vi "generate var cluster.vi"(8 "speed divider":dbl=1.0, 11 "Units":string(combo)) -> (0 "numarray":dbl[](array[numeric]), 1 "varnames":string[](array[string]), 2 "totarray":string[](array[string]), 3 "varclusterarray":T1(array[cluster]))   [LabVIEW 2017]
panel:
  out "Power":dbl[](array[numeric])
  out "appended array":dbl[](array[numeric])
  out "array w/ subset deleted":dbl[](array[numeric])
  out "String Array From File":string[][](array[string])
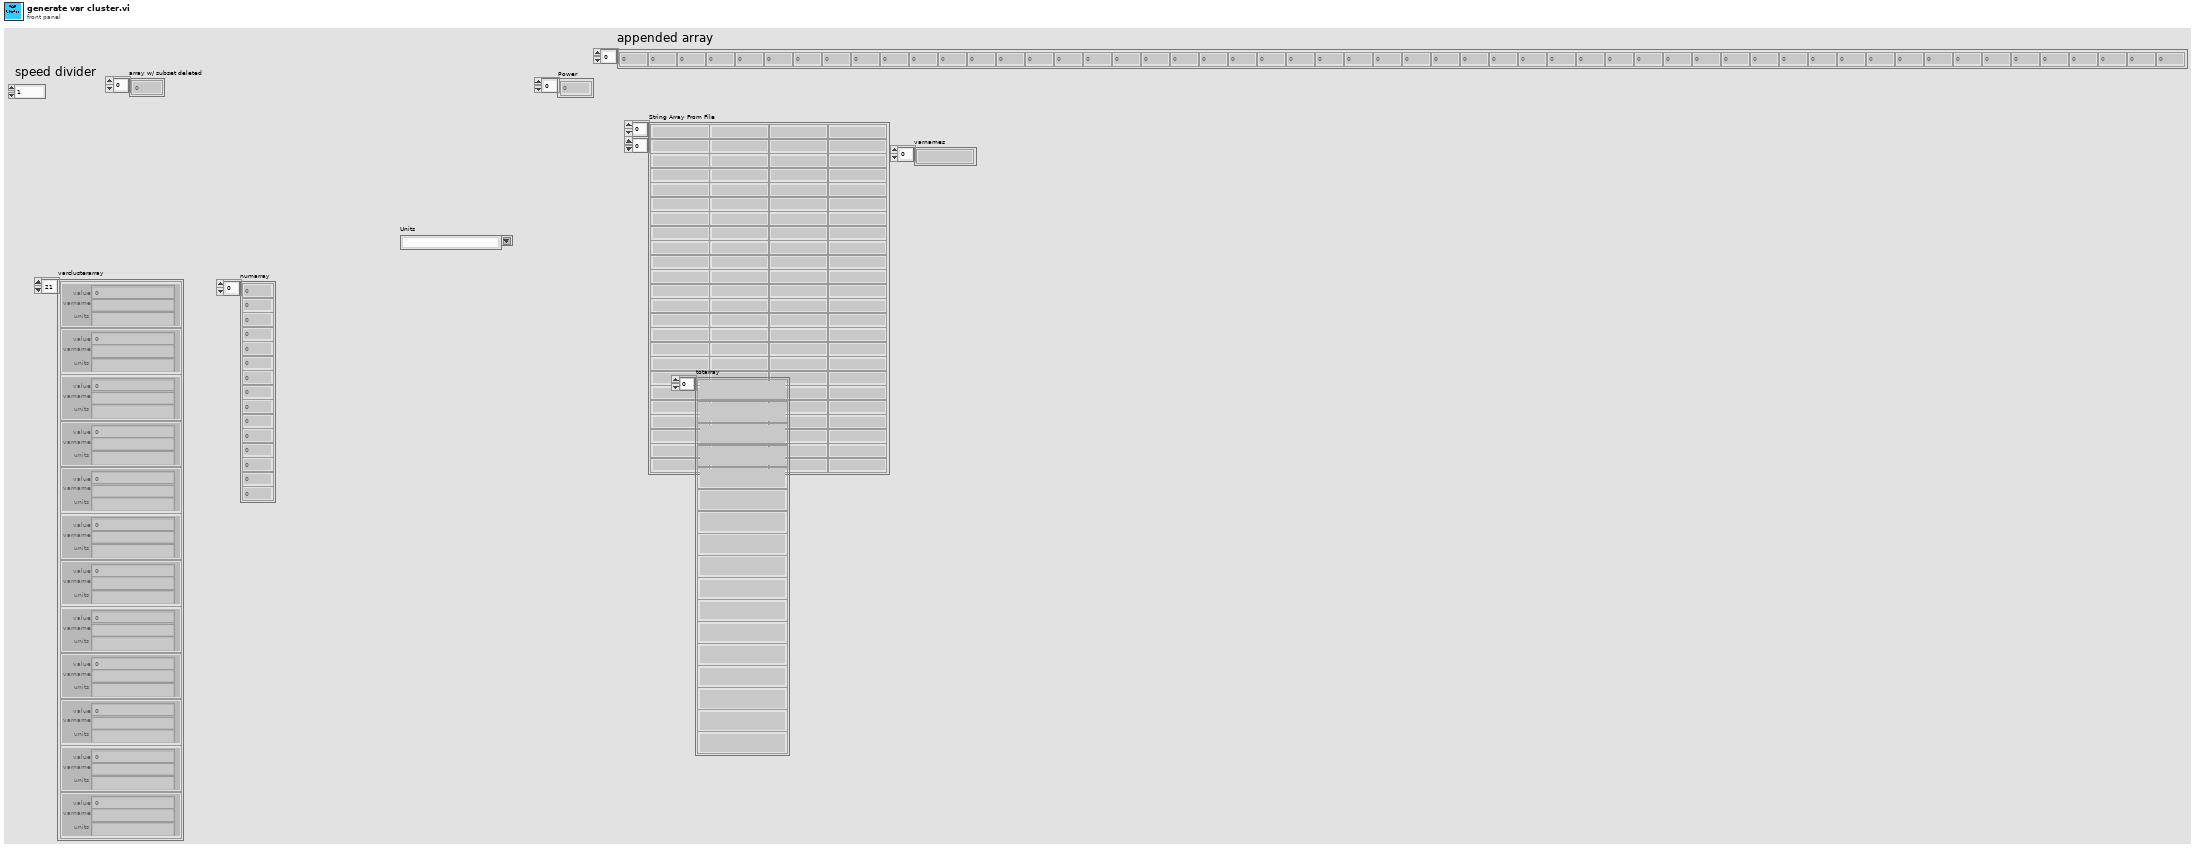
[diagram p1: front panel]
types:
  T1 = cluster{"value":dbl, "varname":string, "units":string}[]
  T2 = cluster{"RTDs":dbl[], "Thermocouples":dbl[], "Pressure Transducers":dbl[], "Mass Flow Meters":dbl[], "Barometer":dbl[], "Accelerometer":dbl[], "Power":dbl[], "Water Valve Position":dbl[]}
  T3 = cluster{"element":dbl, "String":string, "String":string}
  T4 = cluster{"element":dbl, "String":string, "String":string}[]
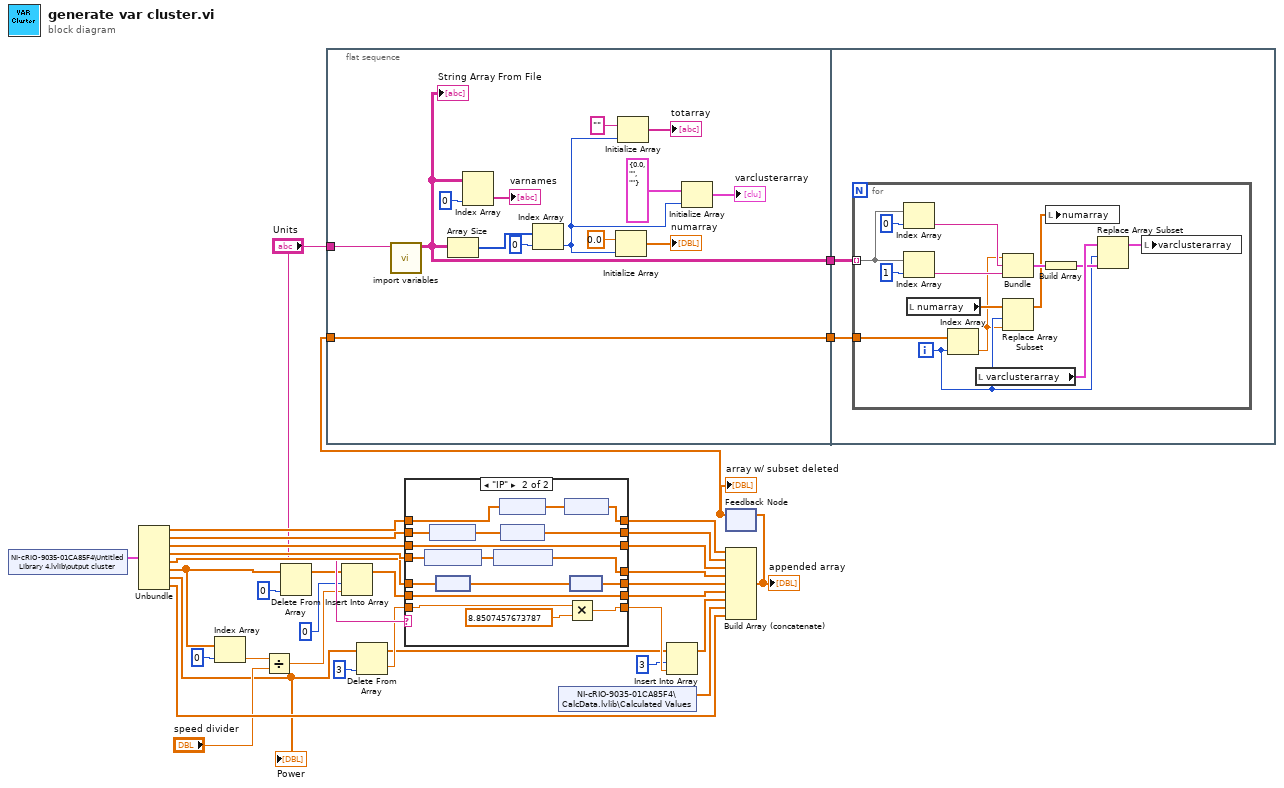
[diagram p0: block diagram]
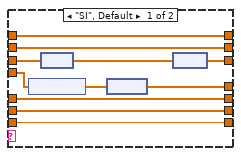
[diagram p2: hidden frame]
diagram:
  n1 = shared-variable "NI-cRIO-9035-01CA85F4\\Untitled Library 4.lvlib\\output cluster"() -> (w18:T2)  [unwired: 1 in, 1 out]
  n2 = Unbundle(w18) -> ("RTDs"=w31:dbl[], "Thermocouples"=w30:dbl[], "Pressure Transducers"=w29:dbl[], "Mass Flow Meters"=w28:dbl[], "Barometer"=w27:dbl[], "Accelerometer"=w9:dbl[], "Power"=w7:dbl[], "Water Valve Position"=w17:dbl[])
  "Power" <- w7
  n3 = Index Array(array=w9, index=0) -> (element=w15:dbl)
  n4 = Divide(x=w15, y="speed divider") -> (x/y=w13:dbl)
  n5 = Delete From Array(array=w9, index=0) -> (array with subset deleted=w8:dbl[])  [unwired: 1 in, 1 out]
  n6 = flat-sequence {
    tunnel: w35 -> [w49]
    tunnel: [w49] -> w34
    tunnel: [w47] -> w33
    tunnel: "Units" -> [w36]
    tunnel: w34 -> [w51]
    tunnel: w33 -> [w50]
    frame #0 {
      n7 = call "import variables.vi"("units"=w36) -> ("String Array From File"=w47:string[][])  [unwired: 9 in, 1 out]
      "String Array From File" <- w47
      n8 = Array Size(array=w47) -> (size(s)=w42:i32[])
      n9 = Index Array(array=w47, index (col)=0 ("disabled index (col)")) -> (element=→"varnames":string[])  [unwired: 1 in]
      n10 = Index Array(array=w42, index=0) -> (element=w45:i32)
      n11 = Initialize Array(0.0, w45) -> (→"numarray":dbl[])
      n12 = Initialize Array("", w45) -> (→"totarray":string[])
      n13 = Initialize Array(cluster{dbl, string, string} {0.0, "", ""}, w45) -> (→"varclusterarray":cluster{dbl, string, string}[])
    }
    frame #1 {
      n14 = for {
        tunnel: w51 -> [w55]
        tunnel: w50 -> [w63] mode=indexing
        i -> [w56]
        n15 = Index Array(array=w63, index=0) -> (element=w64:string)
        n16 = Index Array(array=w63, index=1) -> (element=w61:string)
        n17 = local read "numarray"() -> (w59:dbl[])
        n18 = Index Array(array=w55, index=w56) -> (element=w52:dbl)
        n19 = local read "varclusterarray"() -> (w60:T1)
        n20 = Bundle("element"=w52, "String"=w64, "String"=w61) -> (w58:T3)  [unwired: 1 in]
        n21 = Replace Array Subset(array=w59, new element=w52, index=w56) -> (w53:dbl[])
        n22 = local write "numarray"(w53) -> ()
        n23 = Build Array(w58) -> (w57:T4)
        n24 = Replace Array Subset(array=w60, new element=w57, index=w56) -> (w54:T1)
        n25 = local write "varclusterarray"(w54) -> ()
      }
    }
  }
  n26 = Insert Into Array(array=w8, index=0, new element=w13) -> (w11:dbl[])
  n27 = Delete From Array(array=w7, index=3) -> (deleted portion=w5:dbl, array with subset deleted=w2:dbl[])  [unwired: 1 in]
  n28 = case shown="\"IP\"" "Units" {
    tunnel: w31 -> [w76 w89]
    tunnel: [w76 w90] -> w26
    tunnel: w30 -> [w73 w87]
    tunnel: [w73 w86] -> w25
    tunnel: w29 -> [w71 w93]
    tunnel: [w70 w93] -> w24
    tunnel: w28 -> [w67 w80]
    tunnel: [w68 w81] -> w23
    tunnel: w27 -> [w74 w83]
    tunnel: [w74 w84] -> w22
    tunnel: w11 -> [w75 w92]
    tunnel: [w75 w92] -> w21
    tunnel: w5 -> [w69 w79]
    tunnel: [w69 w77] -> w4
    frame "SI", Default {
      n29 = node(w67) -> (w66:dbl[unit][])
      n30 = node(w71) -> (w72:dbl[unit][])
      n31 = node(w66) -> (w68:dbl[])
      n32 = node(w72) -> (w70:dbl[])
    }
    frame "IP" {
      n33 = node(w80) -> (w82:dbl[unit][])
      n34 = node(w87) -> (w88:dbl[unit][])
      n35 = node(w83) -> (w85:dbl[unit][])
      n36 = node(w82) -> (w81:dbl[])
      n37 = node(w89) -> (w91:dbl[unit][])
      n38 = node(w88) -> (w86:dbl[])
      n39 = node(w91) -> (w90:dbl[])
      n40 = Multiply(x=w79, y=8.8507457673787) -> (x*y=w77:dbl)
      n41 = node(w85) -> (w84:dbl[])
    }
  }
  n42 = shared-variable "NI-cRIO-9035-01CA85F4\\CalcData.lvlib\\Calculated Values"() -> (w32:dbl[])  [unwired: 1 in, 1 out]
  n43 = Insert Into Array(array=w2, index=3, new element=w4) -> (w1:dbl[])
  n44 = feedback #1() -> (w35:dbl[])  [unwired: 1 in]
  "array w/ subset deleted" <- w35
  n45 = Build Array (concatenate)(w26, w25, w24, w23, w22, w21, w1, w32, w17) -> (w19:dbl[])
  "appended array" <- w19
  n46 = feedback-in #1(w19) -> ()
